vi "Write Line.vi"(7 "Output (StdOut)":T1, 8 "error in (no error)":errorcluster, 10 "Text to Write":string, 11 "CLI in":refnum<class "CLI.lvclass">) -> (0 "error out":errorcluster, 3 "CLI out":refnum<class "CLI.lvclass">)   [LabVIEW 2015, in "CLI.lvclass"]
doc: "Write message to output terminated with a line break."
uses:
  CLI.lvclass
  Output.ctl
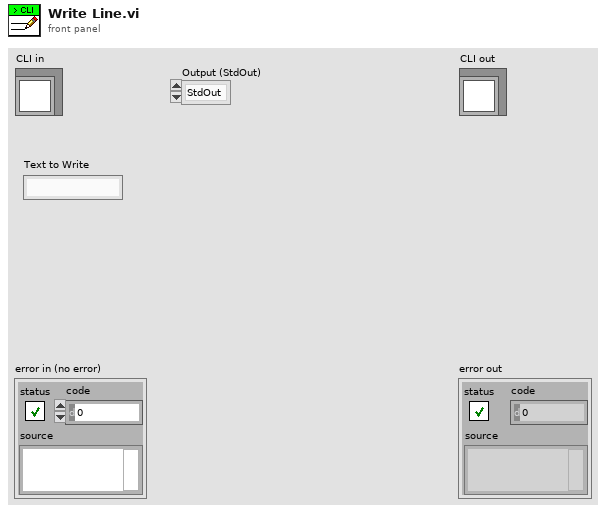
[diagram p1: front panel]
types:
  T1 = typedef "CLI.lvclass/Output.ctl" = enum16{"StdOut", "StdErr"}
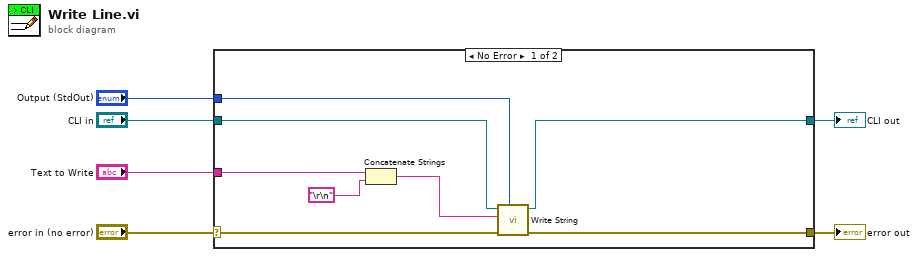
[diagram p0: block diagram]
diagram:
  n1 = case shown="No Error" "error in (no error)" {
    selector: "error in (no error)" -> [w14 w16]
    tunnel: [w13 w16] -> w5
    tunnel: [w11 w15] -> w3
    tunnel: "CLI in" -> [w12 w15]
    tunnel: "Text to Write" -> [w10 _]
    tunnel: "Output (StdOut)" -> [w7 _]
    frame No Error {
      n2 = Concatenate Strings(w10, "\r\n") -> (w9:string)
      n3 = call "Write String.vi"("Output (StdOut)"=w7, "error in (no error)"=w14, "Text to Write"=w9, "CLI in"=w12) -> ("error out"=w13:errorcluster, "CLI out"=w11:refnum<class "CLI.lvclass">)  [unwired: 6 in]
    }
    frame Error {
    }
  }
  "error out" <- w5
  "CLI out" <- w3
